vi "Debug Exercise (Sub).vi"(1 "Number":dbl format="%.2f") -> (0 "Final Result":dbl format="%.2f")   [LabVIEW 2010]
doc: "This VI is the subVI for Exercise 2-3 of the LabVIEW Basics I Course."
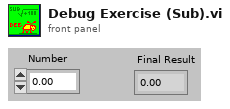
[diagram p1: front panel]
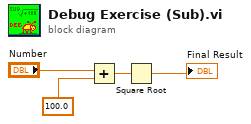
[diagram p0: block diagram]
diagram:
  n1 = Add(x="Number", y=100.0) -> (x+y=w1:dbl)
  n2 = Square Root(x=w1) -> (sqrt(x)=→"Final Result":dbl)
